vi "2020-LoaderMotor.vi"(8 "error in":errorcluster, 11 "Boolean":bool) -> (0 "error out":errorcluster, 3 "Loader Stator Current":dbl)   [LabVIEW 2019]
uses:
  2020LabView/Robot Global Data.vi
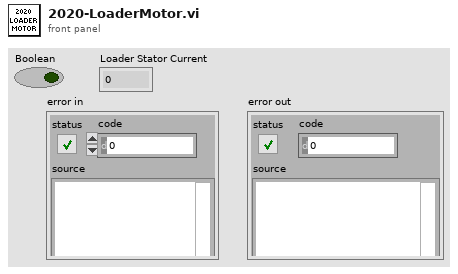
[diagram p1: front panel]
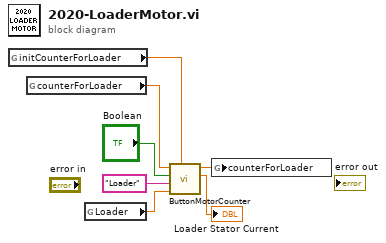
[diagram p0: block diagram]
diagram:
  n1 = global read "Robot Global Data.vi" "initCounterForLoader"() -> (w6:dbl)
  n2 = global read "Robot Global Data.vi" "counterForLoader"() -> (w3:dbl)
  n3 = global read "Robot Global Data.vi" "Loader"() -> (w5:dbl)
  n4 = call "ButtonMotorCounter.vi"("counterStartValue"=w6, "Motor Set Point"=w5, "refnum name"="Loader", "Boolean"="Boolean", "counterForIntake in"=w3) -> ("Stator Current"=→"Loader Stator Current":dbl, "counterForIntake out"=w1:dbl)  [unwired: 5 in]
  n5 = global write "Robot Global Data.vi" "counterForLoader"(w1) -> ()
